vi "get_all_intensity.vi"(8 "Error In":errorcluster, 10 "Sample":string, 11 "File Path":path) -> (0 "Error Out":errorcluster)   [LabVIEW 2019]
uses:
  <vilib>/vision/NI_Vision_Development_Module.lvlib
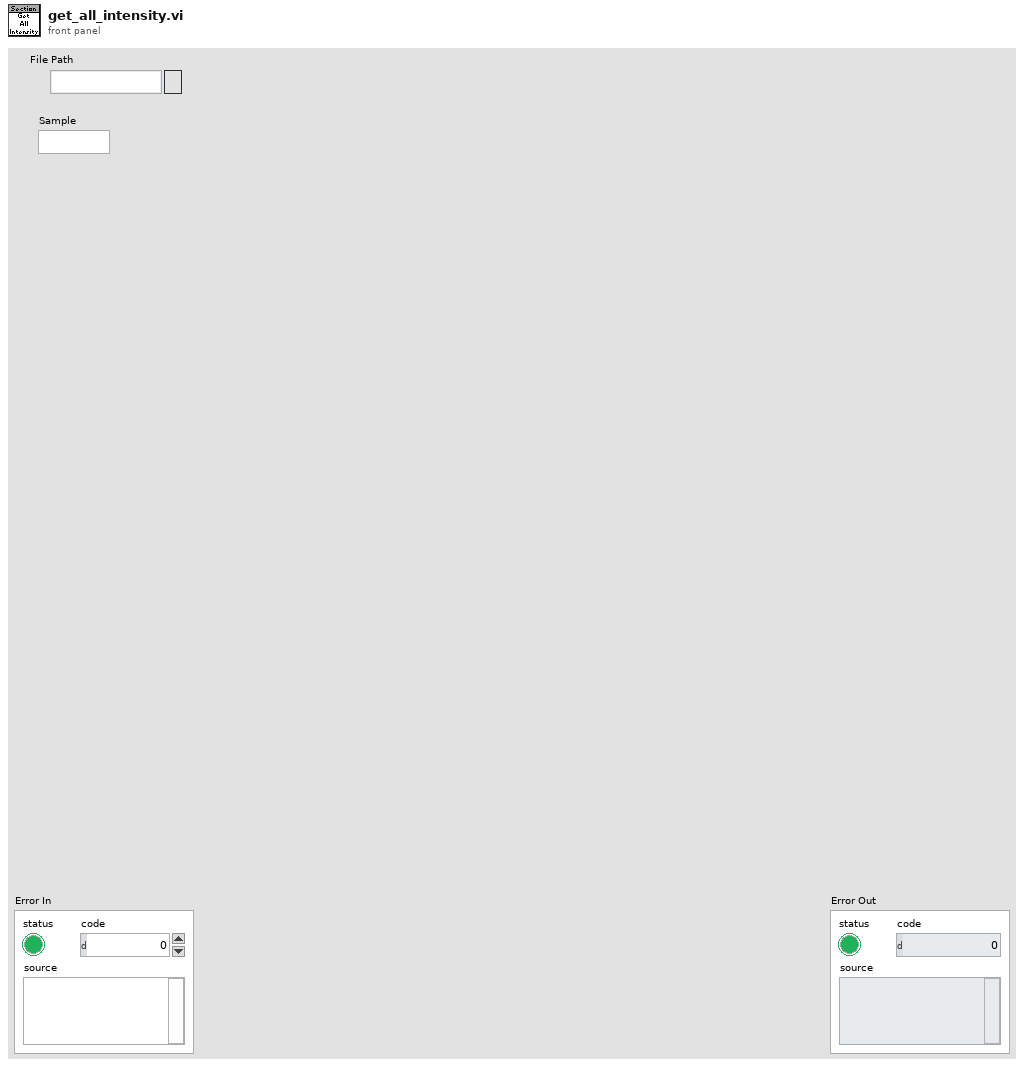
[diagram p1: front panel]
types:
  T1 = typedef "sample_results_cluster_typedef.ctl" = cluster{"File Path":string, "Sample":string, "Threshold":dbl, "Parameters":T2, "Writeable Parameters":T3, "Gain Results":T4[]}
  T2 = typedef "parameters_cluster_typedef.ctl" = cluster{"m1":dbl, "m2":dbl, "m3":dbl, "c":dbl, "D":dbl, "Beta":dbl, "center x":dbl, "center y":dbl}
  T3 = typedef "writeable_section_parameters_cluster_typedef.ctl" = cluster{"Section":string, "Method":i32, "Edge Mode":i32, "Grid Constant":i32, "Manual Sequence":i32, "ROI Size":i32, "Min Grain Size":dbl, "Comments":string, "File Path":string}
  T4 = typedef "grain_results_cluster_typedef.ctl" = cluster{"Grain Number":i32, "xi":dbl[], "phiin":dbl[], "Intensity":dbl[][], "Best Fit Intensity":dbl[][], "Best Fit Parameters":dbl[][], "Polarizer 1 Angle":dbl[][], "Polarizer 2 Angle":dbl[][], "Best Extinction Angle":dbl[], "Best Extinction Angle Corrected":dbl[], "Thetac":dbl, "Phic":dbl, "ROI":cluster{"Global Rectangle":i32[], "Contours":cluster{"Contour Type":u32, "ROI Type":u32, "Points":i32[]}[]}, "a":dbl, "b":dbl, "sequences available":dbl, "sequences used":dbl, "Contrast":dbl[], "Rsq":dbl}
  T5 = typedef "IMAQ Image.ctl" = refnum<image>
  T6 = cluster{"Global Rectangle":i32[], "Contours":cluster{"Contour Type":u32, "ROI Type":u32, "Points":i32[]}[]}
  T7 = typedef "image_property_cluster_typedef.ctl" = cluster{"Stage Angle":dbl, "Sample Angle":dbl, "Polarizer 1 Angle":dbl, "Polarizer 2 Angle":dbl, "Sample Name":string}
  T8 = cluster{"Mean Value":sgl, "Standard Variation":sgl, "Minimal Value":sgl, "Maximal Value":sgl, "Area (calibrated)":sgl, "Area (pixels)":u32, "%":sgl, "Calibration Valid":bool}
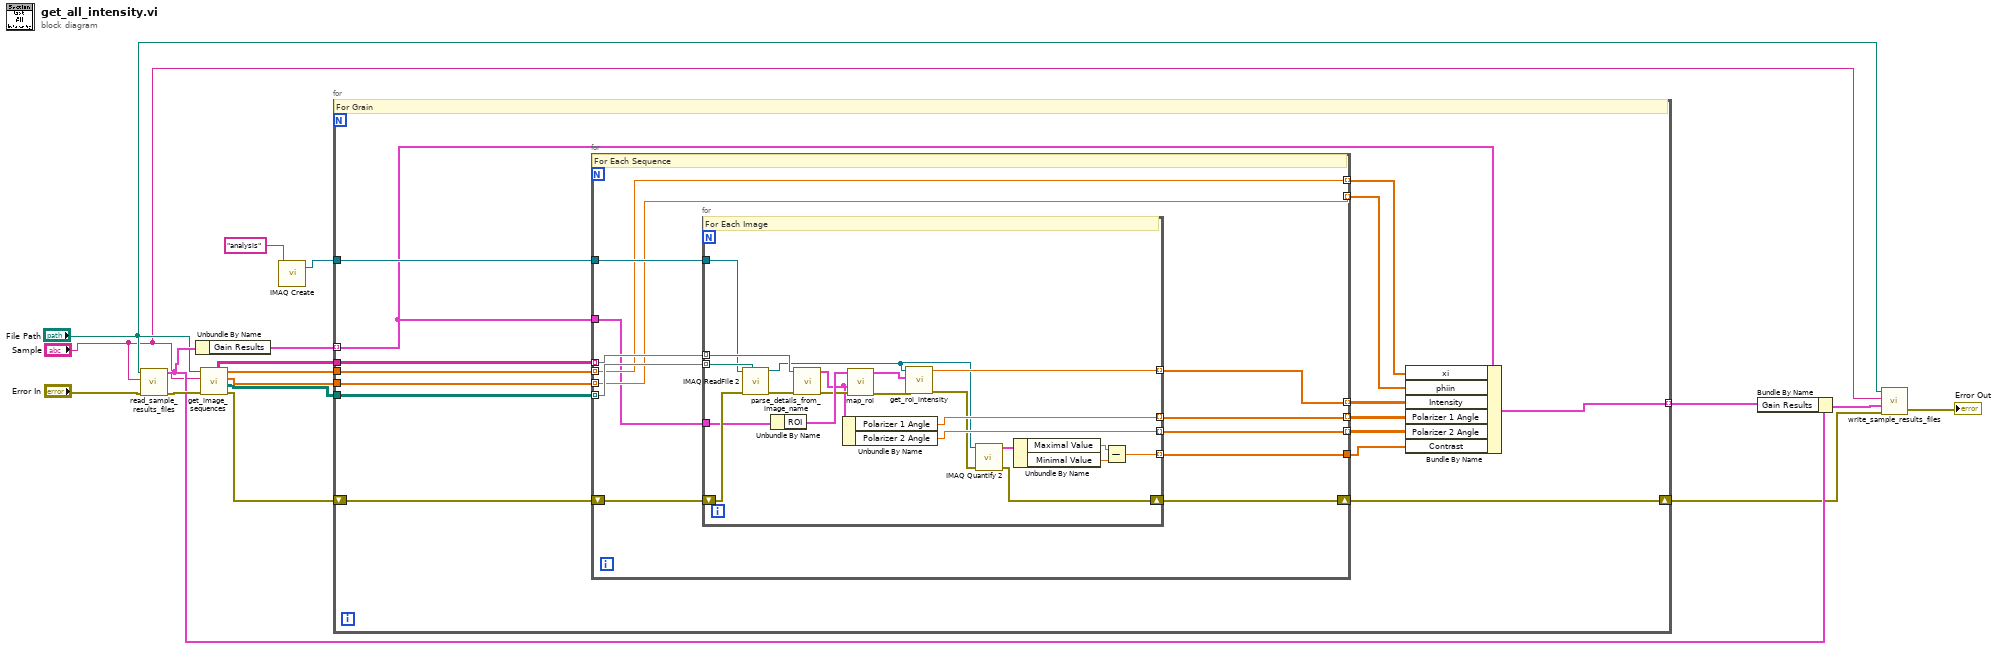
[diagram p0: block diagram]
diagram:
  n1 = call "read_sample_results_files.vi"("Error In"="Error In", "Sample"="Sample", "File Path"="File Path") -> ("Error Out"=w13:errorcluster, "Sample Results"=w7:T1)  [unwired: 7 in]
  n2 = Unbundle By Name(w7) -> ("Gain Results"=w14:T4[])
  n3 = call "get_image_sequences.vi"("Error In"=w13, "Sample"="Sample", "File Path"="File Path") -> ("Error Out"=w12:errorcluster, "File Paths"=w9:path[][], "Phiin"=w10:dbl[], "Xi"=w11:dbl[], "Image Names"=w8:string[][])  [unwired: 4 in]
  n4 = call "IMAQ Create"("Image Name"="analysis") -> ("New Image"=w15:T5)  [unwired: 4 in, 1 out]
  n5 = for {
    tunnel: w15 -> [w27]
    shift-right: [w21] -> w2
    shift-left: w12 -> [w32]
    tunnel: w14 -> [w19] mode=indexing
    tunnel: w11 -> [w31]
    tunnel: w10 -> [w30]
    tunnel: w9 -> [w29]
    tunnel: w8 -> [w28]
    tunnel: [w20] -> w6 mode=indexing
    # "For Grain"
    n6 = for {
      shift-right: [w35] -> w21
      shift-left: w32 -> [w44]
      tunnel: w31 -> [w40] mode=indexing
      tunnel: w30 -> [w39] mode=indexing
      tunnel: w29 -> [w43] mode=indexing
      tunnel: w28 -> [w42] mode=indexing
      tunnel: w27 -> [w41]
      tunnel: [w40] -> w26 mode=indexing
      tunnel: [w39] -> w25 mode=indexing
      tunnel: [w38] -> w24 mode=indexing
      tunnel: [w37] -> w23 mode=indexing
      tunnel: [w36] -> w22 mode=indexing
      tunnel: w19 -> [w34]
      tunnel: [w33] -> w18
      # "For Each Sequence"
      n7 = for {
        shift-right: [w49] -> w35
        shift-left: w44 -> [w65]
        tunnel: [w59] -> w38 mode=indexing
        tunnel: w43 -> [w58] mode=indexing
        tunnel: w42 -> [w57] mode=indexing
        tunnel: w41 -> [w56]
        tunnel: [w54] -> w37 mode=indexing
        tunnel: [w53] -> w36 mode=indexing
        tunnel: w34 -> [w52]
        tunnel: [w45] -> w33 mode=indexing
        # "For Each Image"
        n8 = call "IMAQ ReadFile 2"("File Path"=w58, "error in (no error)"=w65, "Image"=w56) -> ("error out"=w64:errorcluster, "Image Out"=w51:T5)  [unwired: 4 in, 3 out]
        n9 = Unbundle By Name(w52) -> ("ROI"=w63:T6)
        n10 = call "parse_details_from_image_name.vi"("Error In"=w64, "Image Name"=w57) -> ("Error Out"=w62:errorcluster, "Image Properties"=w55:T7)  [unwired: 8 in]
        n11 = Unbundle By Name(w55) -> ("Polarizer 1 Angle"=w54:dbl, "Polarizer 2 Angle"=w53:dbl)
        n12 = call "map_roi.vi"("Error In"=w62, "Image Properties"=w55, "ROI In"=w63) -> ("Error Out"=w60:errorcluster, "ROI Out"=w61:T6)  [unwired: 7 in]
        n13 = call "get_roi_intensity.vi"("Error In"=w60, "ROI In"=w61, "Image"=w51) -> ("Error Out"=w50:errorcluster, "Intensity"=w59:dbl)  [unwired: 7 in]
        n14 = call "IMAQ Quantify 2"("error in (no error)"=w50, "Image"=w51) -> ("error out"=w49:errorcluster, "Global Report"=w48:T8)  [unwired: 7 in, 1 out]
        n15 = Unbundle By Name(w48) -> ("Maximal Value"=w46:sgl, "Minimal Value"=w47:sgl)
        n16 = Subtract(x=w46, y=w47) -> (x-y=w45:sgl)
      }
    }
    n17 = Bundle By Name(cluster=w19, "xi"=w26, "phiin"=w25, "Intensity"=w24, "Polarizer 1 Angle"=w23, "Polarizer 2 Angle"=w22, "Contrast"=w18) -> (w20:T4)
  }
  n18 = Bundle By Name(cluster=w7, "Gain Results"=w6) -> (w5:T1)
  n19 = call "write_sample_results_files.vi"("Error In"=w2, "Sample Results"=w5, "Sample"="Sample", "File Path"="File Path") -> ("Error Out"=→"Error Out":errorcluster)  [unwired: 7 in]
